vi "Initialize.vi"(7 "Serial Configuration":T1={"Baud Rate"=115200, "Parity"=0, "Data Bits"=8, "Stop Bits"=10, "Flow Control"=0} {"Flow Control" items=["None", "XON/XOFF", "RTS/CTS", "XON/XOFF & RTS/CTS", "DTR/DSR", "XON/XOFF & DTR/DSR"]; "Stop Bits" items=["1.0"=10, "1.5"=15, "2.0"=20]; "Data Bits" items=["7"=7, "8"=8]; "Parity" items=["None", "Odd", "Even", "Mark", "Space"]; "Baud Rate" items=["300"=300, "600"=600, "1200"=1200, "2400"=2400, "4800"=4800, "9600"=9600, "19200"=19200]}, 8 "error in (no error)":errorcluster, 9 "Reset (True)":bool, 10 "ID Query (True)":bool=TRUE, 11 "VISA resource name":refnum<visa-resource-name>) -> (0 "error out":errorcluster, 3 "VISA resource name out":refnum<visa-resource-name>)   [LabVIEW 2014, in "GRBLMotionCore.lvlib"]
doc: "Establishes communication with the instrument and optionally performs an instrument identification query and/or an instrument reset. It also places the instrument in a default state needed for other instrument driver operations. Therefore, call this VI before calling other instrument driver VIs for this instrument. Generally, you need to call the Initialize VI only once at the beginning of an application."
uses:
  <instrlib>/GRBL/GRBLMotionCore.lvlib
panel:
  # "(c) 2007 <Enter Company Name Here>.  ALL RIGHTS RESERVED."
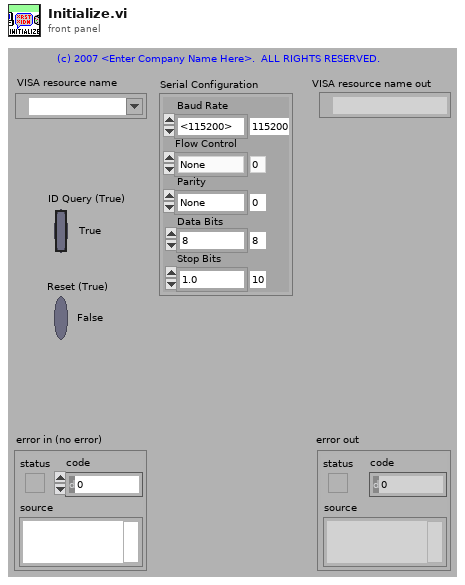
[diagram p1: front panel]
types:
  T1 = cluster{"Baud Rate":u32, "Parity":u16, "Data Bits":u16, "Stop Bits":u16, "Flow Control":u16}
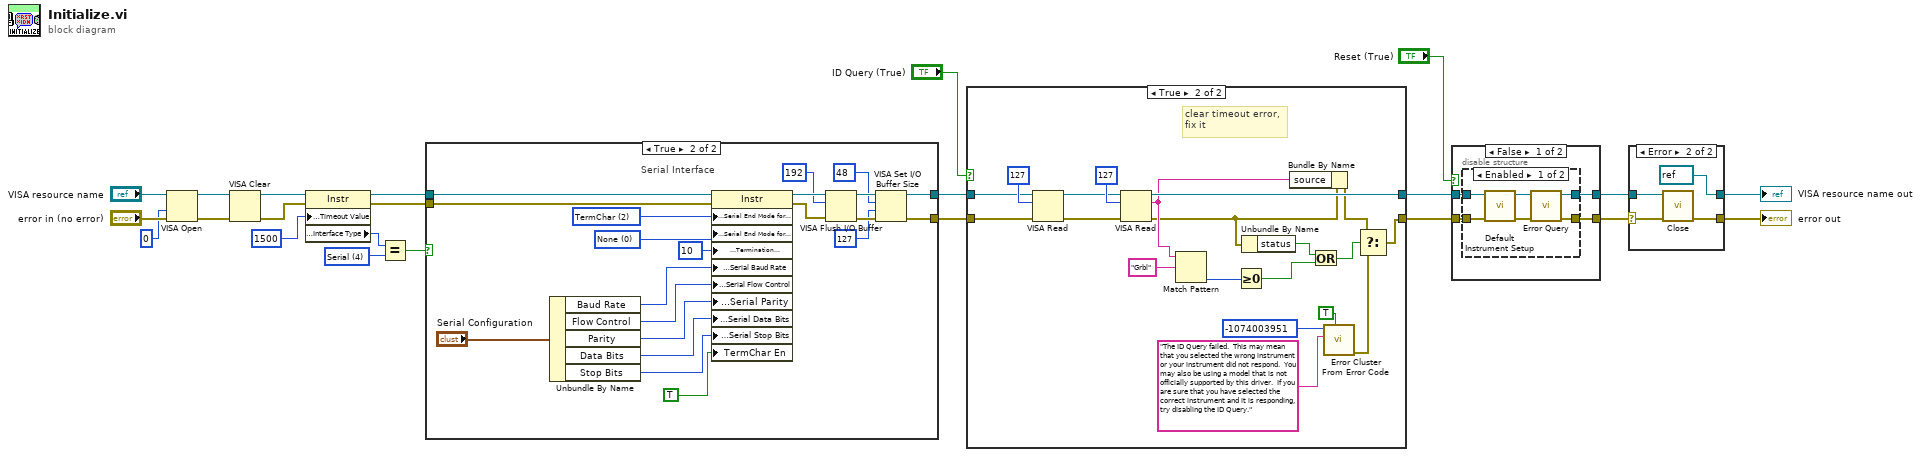
[diagram p0: block diagram]
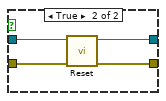
[diagram p5: hidden frame]
diagram:
  w10 = u16 4 items=["GPIB"=1, "VXI"=2, "GPIB-VXI"=3, "Serial"=4, "PXI"=5, "TCPIP"=6, "USB"=7] ("Interface Information:Interface Type")
  n1 = VISA Open(access mode=u32 0, error in (no error)="error in (no error)", VISA resource name="VISA resource name") -> (VISA resource name=w8:refnum<visa-resource-name>, error out=w7:errorcluster)  [unwired: 2 in]
  n2 = VISA Clear(VISA resource name=w8, error in (no error)=w7) -> (VISA resource name out=w6:refnum<visa-resource-name>, error out=w5:errorcluster)
  n3 = property class="Instr"(reference=w6, error in=w5, "General Settings:Timeout Value"=u32 1500) -> (reference out=w13:refnum<visa-resource-name>, error out=w12:errorcluster, "Interface Information:Interface Type"=w17:u16)
  n4 = Equal?(x=w17, y=w10) -> (x = y?=w11:bool)
  n5 = case shown="True" w11 {
    tunnel: [w24 w43] -> w15
    tunnel: [w25 w40] -> w14
    tunnel: w13 -> [w24 w45]
    tunnel: w12 -> [w25 w46]
    frame False {
      # "EDIT: Remove interfaces not\nsupported by your instrument."
      # "GPIB, TCP/IP, and USB Interface"
    }
    frame True {
      w26 = u16 0 items=["None", "Last Bit", "TermChar", "Break"] ("Serial Settings:End Mode for Writes")
      w35 = u16 2 items=["None", "LastBit", "TermChar"] ("Serial Settings:Serial End Mode for Reads")
      # "Serial Interface"
      n6 = Unbundle By Name("Serial Configuration") -> ("Baud Rate"=w34:u32, "Flow Control"=w30:u16, "Parity"=w32:u16, "Data Bits"=w33:u16, "Stop Bits"=w29:u16)
      n7 = property class="Instr"(reference=w45, error in=w46, "Serial Settings:Serial End Mode for Reads"=w35, "Serial Settings:Serial End Mode for Writes"=w26, "Message Based Settings:Termination Character"=u8 10, "Serial Settings:Serial Baud Rate"=w34, "Serial Settings:Serial Flow Control"=w30, "Serial Settings:Serial Parity"=w32, "Serial Settings:Serial Data Bits"=w33, "Serial Settings:Serial Stop Bits"=w29, "TermChar En"=TRUE ("Message Based Settings:Termination Character Enable")) -> (reference out=w39:refnum<visa-resource-name>, error out=w42:errorcluster)
      n8 = VISA Flush I/O Buffer(VISA resource name=w39, mask (16)=u16 192, error in (no error)=w42) -> (VISA resource name out=w44:refnum<visa-resource-name>, error out=w41:errorcluster)
      n9 = VISA Set I/O Buffer Size(VISA resource name=w44, mask (16)=u16 48, size (4096)=u32 127 ("size (0)"), error in (no error)=w41) -> (VISA resource name out=w43:refnum<visa-resource-name>, error out=w40:errorcluster)
    }
  }
  n10 = case shown="True" "ID Query (True)" {
    tunnel: [w47 w68] -> w22
    tunnel: [w48 w67] -> w23
    tunnel: w15 -> [w48 w50]
    tunnel: w14 -> [w47 w51]
    frame False {
    }
    frame True {
      # "clear timeout error,\nfix it"
      n11 = VISA Read(VISA resource name=w50, byte count=u32 127, error in (no error)=w51) -> (VISA resource name out=w53:refnum<visa-resource-name>, error out=w52:errorcluster)  [unwired: 2 out]
      n12 = VISA Read(VISA resource name=w53, byte count=u32 127, error in (no error)=w52) -> (VISA resource name out=w67:refnum<visa-resource-name>, read buffer=w56:string, error out=w55:errorcluster)  [unwired: 1 out]
      n13 = Match Pattern(string=w56, regular expression="Grbl") -> (offset past match=w61:i32)  [unwired: 1 in, 3 out]
      n14 = Greater Or Equal To 0?(x=w61) -> (x >= 0?=w49:bool)
      n15 = Unbundle By Name(w55) -> ("status"=w60:bool)
      n16 = Bundle By Name(cluster=w55, "source"=w56) -> (w57:errorcluster)
      n17 = Or(x=w60, y=w49) -> (x .or. y?=w59:bool)
      n18 = call <vilib>:"Error Cluster From Error Code.vi"("show call chain? (False)"=TRUE, "error message (\"\")"="The ID Query failed.  This may mean that you selected the wrong instrument or your instrument did not respond.  You may also be using a model that is not officially supported by this driver.  If you are sure that you have selected the correct instrument and it is responding, try disabling the ID Query." ("Source (VI Name)"), "error code (0)"=-1074003951 ("Code")) -> ("error out"=w65:errorcluster)  [unwired: 6 in]
      n19 = Select(t=w57, s=w59, f=w65) -> (s? t:f=w68:errorcluster)
    }
  }
  n20 = case shown="False" "Reset (True)" {
    tunnel: w22 -> [w71 w81]
    tunnel: [w69 w84] -> w1
    tunnel: w23 -> [w72 w82]
    tunnel: [w70 w83] -> w2
    frame False {
      n21 = disable-structure shown="Enabled" {
        disable-tunnel: w72 -> [w78 w80]
        disable-tunnel: w71 -> [w77 w79]
        disable-tunnel: [w76 w80] -> w70
        disable-tunnel: [w75 w79] -> w69
        frame Enabled {
          n22 = call <instrlib>:"Default Instrument Setup.vi"("error in (no error)"=w77, "VISA resource name"=w78) -> ("error out"=w73:errorcluster, "VISA resource name out"=w74:refnum<visa-resource-name>)  [unwired: 8 in]
          n23 = call <instrlib>:"Error Query.vi"("error in (no error)"=w73, "VISA resource name"=w74) -> ("error out"=w75:errorcluster, "VISA resource name out"=w76:refnum<visa-resource-name>)  [unwired: 6 in, 2 out]
        }
        frame Disabled {
        }
      }
    }
    frame True {
      n24 = call <instrlib>:"Reset.vi"("error in (no error)"=w81, "VISA resource name"=w82) -> ("error out"=w84:errorcluster, "VISA resource name out"=w83:refnum<visa-resource-name>)  [unwired: 8 in]
    }
  }
  n25 = case shown="Error" w1 {
    selector: w1 -> [w85 w88]
    tunnel: w2 -> [w86 w89]
    tunnel: [w86 refnum<visa-resource-name> refnum ("VISA resource name out")] -> w4
    tunnel: [w85 w90] -> w3
    frame No Error {
    }
    frame Error {
      n26 = call <instrlib>:"Close.vi"("error in (no error)"=w88, "VISA resource name"=w89) -> ("error out"=w90:errorcluster)  [unwired: 9 in]
    }
  }
  "VISA resource name out" <- w4
  "error out" <- w3
